vi "Close.vi"(8 "error in (no error)":errorcluster, 11 "Data in":refnum<class "UI-Bus.lvclass">) -> (0 "error out":errorcluster, 3 "Data out":refnum<class "UI-Bus.lvclass">)   [LabVIEW 2021, in "UI-Bus.lvclass"]
doc: "Abstract Data Classes 2.1.1.13\nTim Streeter - TSA\nCopyright (c) 2025, TSA"
uses:
  UI-Bus.lvclass
  C:/Program Files (x86)/National Instruments/LabVIEW 2021/vi.lib/TSA/Omni-Bus/Omni-Bus/Bus Access/Bus_Access.lvclass
  <vilib>/TSA/Omni-Bus/Omni-Bus/Bus Access/Bus_Access.lvclass/Bus_Access.ctl
  UI-Bus.lvclass/UI-Bus.ctl
  <vilib>/TSA/Omni-Bus/Omni-Bus/Bus Access/Properties/Read Values.vi
  <vilib>/TSA/Abstract Data Classes/Abs_Types/Type/Abs_Type.lvclass
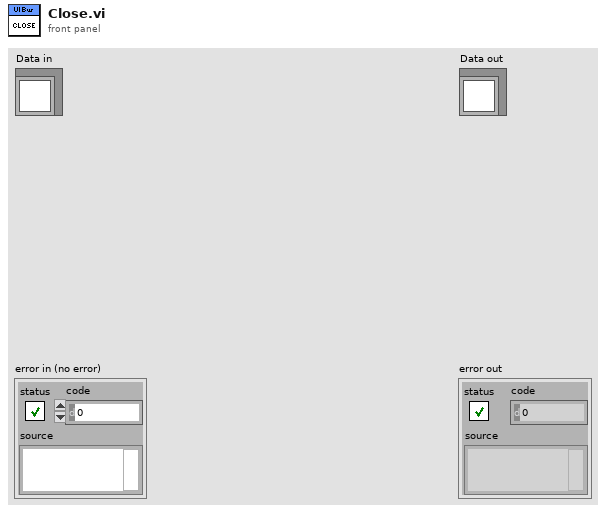
[diagram p1: front panel]
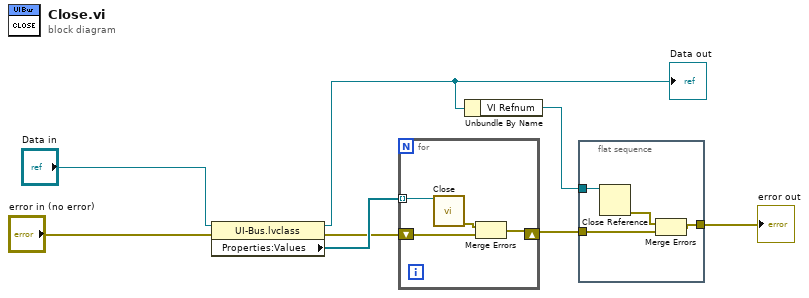
[diagram p0: block diagram]
diagram:
  n1 = property class="UI-Bus.lvclass"(reference="Data in", error in="error in (no error)") -> (reference out=w4:refnum<class "UI-Bus.lvclass">, error out=w7:errorcluster, "Properties:Values"=w8:refnum<class "Abs_Type.lvclass">[])
  "Data out" <- w4
  n2 = for {
    tunnel: w8 -> [w12] mode=indexing
    shift-right: [w10] -> w3
    shift-left: w7 -> [w9]
    n3 = call-dynamic "Close.vi"("Data in"=w12) -> ("error out"=w11:errorcluster)  [unwired: 9 in, 1 out]
    n4 = Merge Errors(w11, w9) -> (w10:errorcluster)
  }
  n5 = Unbundle By Name(w4) -> ("VI Refnum"=w1:refnum<vi>)
  n6 = flat-sequence {
    tunnel: w3 -> [w16]
    tunnel: [w14] -> w2
    tunnel: w1 -> [w13]
    frame #0 {
      n7 = Close Reference(reference=w13) -> (error out=w15:errorcluster)  [unwired: 1 in]
      n8 = Merge Errors(w15, w16) -> (w14:errorcluster)
    }
  }
  "error out" <- w2
